vi "GetPackageList.vi"(8 "error in (no error)":errorcluster, 11 "service":refnum<class "IcmMessageService.lvclass">) -> (0 "error out":errorcluster, 2 "string":string, 3 "service out":refnum<class "IcmMessageService.lvclass">)   [LabVIEW 2016]
doc: "Queries for all equipment asset nodes, which means they have operating states."
uses:
  <vilib>/addons/InsightCM/MessageBus/MessageService/IcmMessageService.lvclass
panel:
  out "output cluster":T1
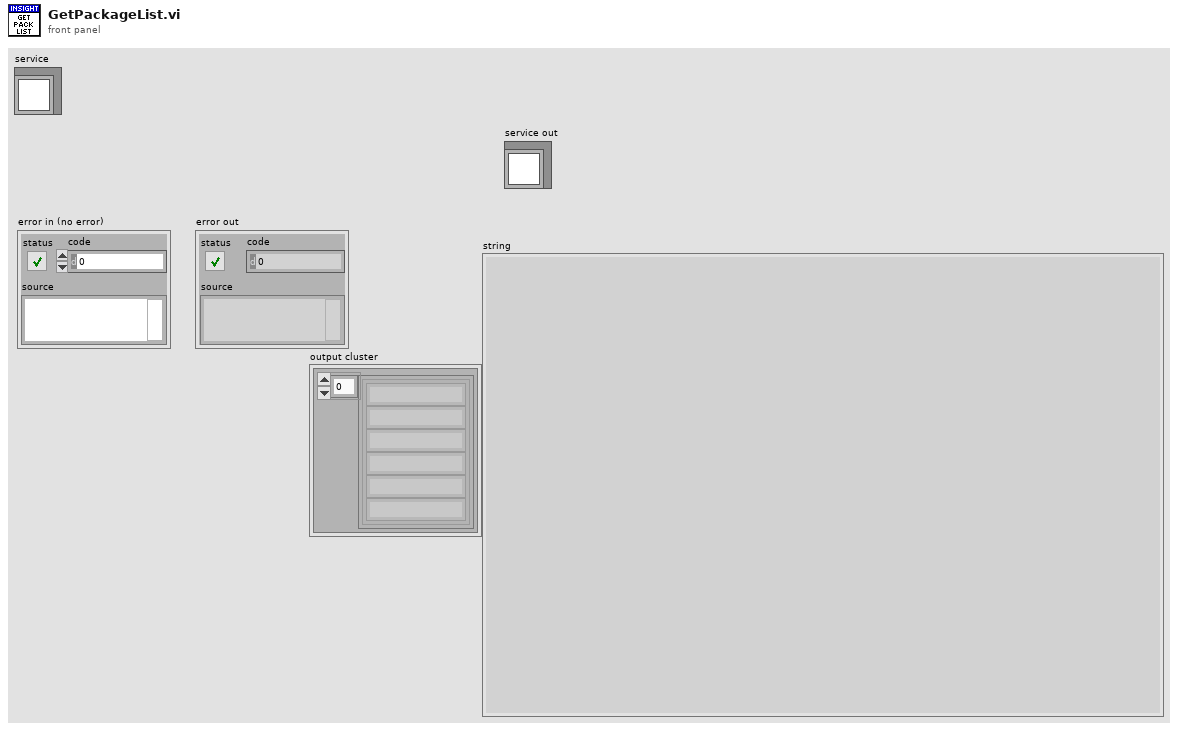
[diagram p1: front panel]
types:
  T1 = cluster{cluster{cluster{string, string, string, string, string, string}[]}}
  T2 = typedef "Message.ctl" = cluster{"Header":T3, "Body":u8[]}
  T3 = typedef "MessageHeader.ctl" = cluster{"MessageName":string, "Timestamp":i64, "CorrelationId":string, "ContentType":string, "RoutingKey":string, "Properties":T4[]}
  T4 = typedef "KeyValuePair.ctl" = cluster{"Key":string, "Value":string}
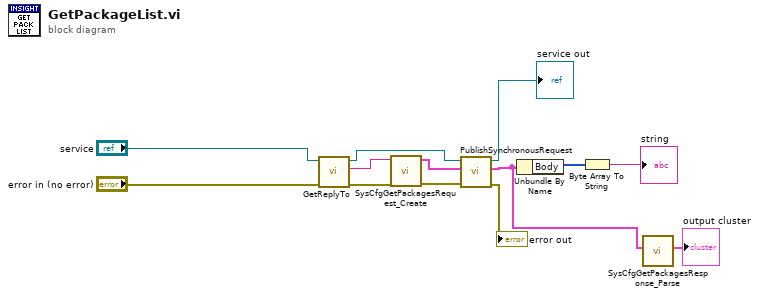
[diagram p0: block diagram]
diagram:
  n1 = call <vilib>:"GetReplyTo.vi"("error in (no error)"="error in (no error)", "service in"="service") -> ("error out"=w7:errorcluster, "reply to"=w8:string, "service out"=w11:refnum<class "IcmMessageService.lvclass">)  [unwired: 7 in]
  n2 = call <vilib>:"SysCfgGetPackagesRequest_Create.vi"("error in (no error)"=w7, "ReplyTo"=w8) -> ("error out"=w6:errorcluster, "Message"=w5:T2)  [unwired: 8 in]
  n3 = call <vilib>:"PublishSynchronousRequest.vi"("error in (no error)"=w6, "request"=w5, "service in"=w11) -> ("error out"=→"error out":errorcluster, "response"=w2:T2, "service out"=→"service out":refnum<class "IcmMessageService.lvclass">)  [unwired: 6 in]
  n4 = Unbundle By Name(w2) -> ("Body"=w10:u8[])
  n5 = Byte Array To String(unsigned byte array=w10) -> (string=→"string":string)
  n6 = call "SysCfgGetPackagesResponse_Parse.vi"("Message"=w2) -> ("output cluster"=→"output cluster":T1)  [unwired: 10 in]
